vi "Calculate Score Of Winner Board.vi"(10 "Winner Board Status":bool[][](array[boolean]), 11 "Winner Board":i32[][](array[numeric])) -> (3 "Score":i32)   [LabVIEW 2019, in "Day 4.lvlib"]
uses:
  Day 4.lvlib
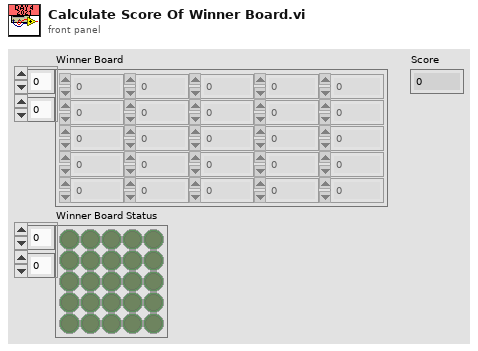
[diagram p1: front panel]
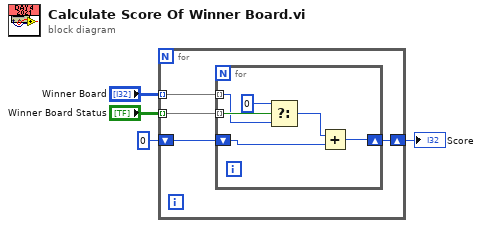
[diagram p0: block diagram]
diagram:
  n1 = for {
    tunnel: "Winner Board" -> [w8] mode=indexing
    tunnel: "Winner Board Status" -> [w7] mode=indexing
    shift-right: [w6] -> w1
    shift-left: 0 -> [w5]
    n2 = for {
      tunnel: w8 -> [w13] mode=indexing
      tunnel: w7 -> [w14] mode=indexing
      shift-right: [w9] -> w6
      shift-left: w5 -> [w10]
      n3 = Select(t=0, s=w14, f=w13) -> (s? t:f=w11:i32)
      n4 = Add(x=w11, y=w10) -> (x+y=w9:i32)
    }
  }
  "Score" <- w1
